vi "TDMS Write Time Domain Data.vi"() -> ()   [LabVIEW 2023]
doc: "Demonstrates how to write time-domain data to a .tdms file with the TDMS Write function."
uses:
  <vilib>/Utility/TDMS File Viewer/NI_TDMS File Viewer.lvlib
panel:
  in  "Title":string="LabVIEW Example (time domain)"
  in  "Stop":bool
  out "Graph":waveform(dbl)[](graph)
  # "Overview: Demonstrates how to write time-domain data to a .tdms file with the TDMS Write function.\nInstructions:\n1. Run the VI.\n2. Click Stop to stop the VI.\n3. Delete the .tdms file (located at [LabVIEW Data]\\Example Time Domain Data.tdms) when you are done."
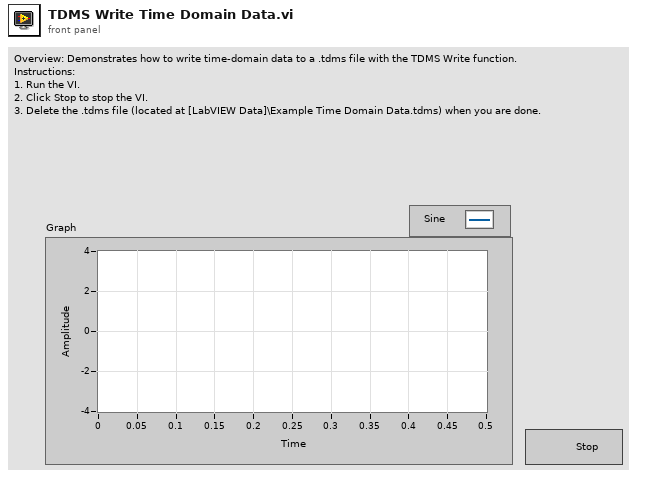
[diagram p1: front panel]
types:
  T1 = enum16{"open", "open or create", "create or replace", "create", "open (read-only)"}
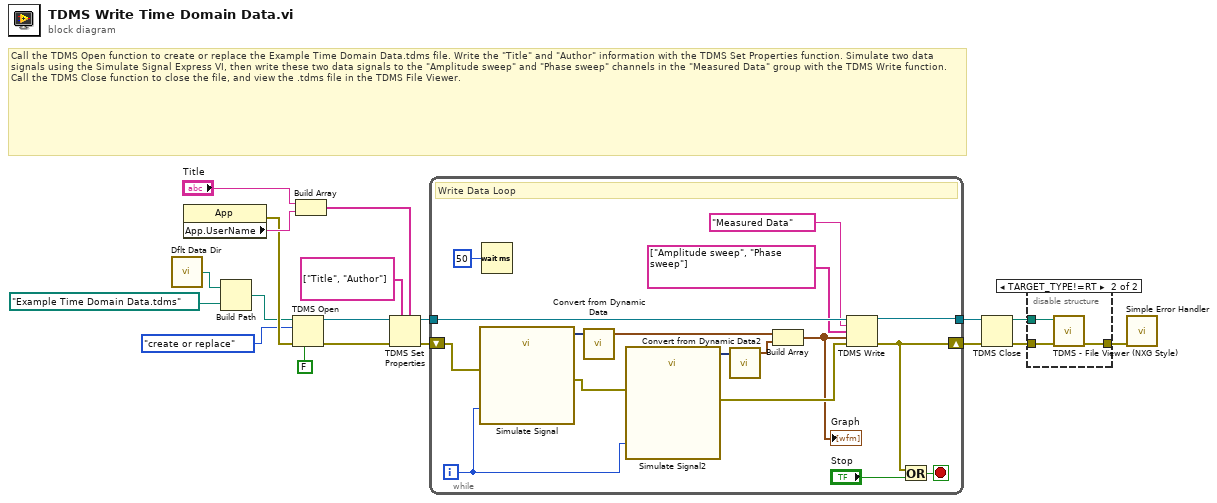
[diagram p0: block diagram]
diagram:
  # "Call the TDMS Open function to create or replace the Example Time Domain Data.tdms file. Write the \"Title\" and \"Author\" information with the TDMS Set Properties function. Simulate two data signals using the Simulate Signal Express VI, then write these two data signals to the \"Amplitude sweep\" and \"Phase sweep\" channels in the \"Measured Data\" group with the TDMS Write function. Call the TDMS Close function to close the file, and view the .tdms file in the TDMS File Viewer."
  n1 = call <vilib>:"Dflt Data Dir.vi"() -> ("App:Default Data Directory"=w19:path)
  n2 = property class="App"() -> (error out=w4:errorcluster, "App.UserName"=w15:string)  [unwired: 2 in, 1 out]
  n3 = Build Path(base path=w19, name or relative path=path "Example Time Domain Data.tdms" ("file path")) -> (appended path=w2:path)
  n4 = TDMS Open(6:FALSE ("disable buffering (T)"), 8:w4, 10:T1."create or replace" ("operation"), 11:w2) -> (0:w17:errorcluster, 3:w18:refnum<k34>)  [unwired: 3 in]
  n5 = Build Array("Title", w15) -> (w14:string[])
  n6 = TDMS Set Properties(5:w14, 7:string[] ["Title", "Author"] ("property names"), 8:w17, 11:w18) -> (0:w13:errorcluster, 3:w12:refnum<k34>)  [unwired: 4 out]
  n7 = while {
    shift-right: [w30] -> w10
    shift-left: w13 -> [w21]
    tunnel: w12 -> [w36]
    tunnel: [w34] -> w11
    i -> [w23]
    stop <- w31 stop-if-true
    # "Write Data Loop"
    n8 = call "Simulate Signal"("Amplitude"=w23, "error in (no error)"=w21) -> ("Sine"=w29:dynamicdata, "error out"=w28:errorcluster)  [unwired: 12 in]
    n9 = Wait (ms)(milliseconds to wait=u32 50) -> ()  [unwired: 1 out]
    n10 = call "Convert from Dynamic Data"("Dynamic Data Type"=w29) -> ("Waveform"=w26:waveform(dbl))  [unwired: 3 in]
    n11 = call "Simulate Signal2"("Phase"=w23, "error in (no error)"=w28) -> ("Sine"=w27:dynamicdata, "error out"=w24:errorcluster)  [unwired: 12 in]
    n12 = call "Convert from Dynamic Data2"("Dynamic Data Type"=w27) -> ("Waveform"=w25:waveform(dbl))  [unwired: 3 in]
    n13 = Build Array(w26, w25) -> (w22:waveform(dbl)[])
    "Graph" <- w22
    n14 = TDMS Write(0:w36, 5:"Measured Data" ("group name"), 7:string[] ["Amplitude sweep", "Phase sweep"] ("channel names"), 9:w22, 11:w24) -> (4:w34:refnum<k34>, 15:w30:errorcluster)  [unwired: 1 in, 2 out]
    n15 = Or(x=w30, y="Stop") -> (x .or. y?=w31:bool)
  }
  n16 = TDMS Close(8:w10, 11:w11) -> (0:w8:errorcluster, 3:w6:path)
  n17 = disable-structure shown="TARGET_TYPE!=RT" {
    disable-tunnel: w8 -> [w37 w40]
    disable-tunnel: w6 -> [_ w39]
    disable-tunnel: [w37 w38] -> w5
    frame condition #0 {
    }
    frame condition #1 (active) {
      n18 = call <vilib>:"TDMS - File Viewer (NXG Style).vi"("error in"=w40, "file in"=w39) -> ("error out"=w38:errorcluster)  [unwired: 8 in, 1 out]
    }
  }
  n19 = call <vilib>:"Simple Error Handler.vi"("error in (no error)"=w5) -> ()  [unwired: 2 in, 7 out]
